vi "aggregator - v - real.vi"(8 "number":dbl, 10 "init?":bool, 11 "requested size":i32=20) -> (1 "Array":dbl[](array[numeric]))   [LabVIEW 2015]
uses:
  agregator -- action.ctl
  linear interpolation - real.vi
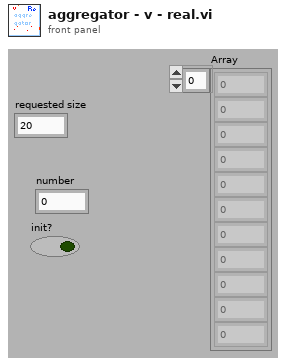
[diagram p1: front panel]
types:
  T1 = typedef "agregator -- action.ctl" = enum16{"append", "interpolate", "empty!", "force"}
  T2 = typedef "interpolation state - real.ctl" = cluster{"requested size":i32, "Array":dbl[], "actual number of elements":i32}
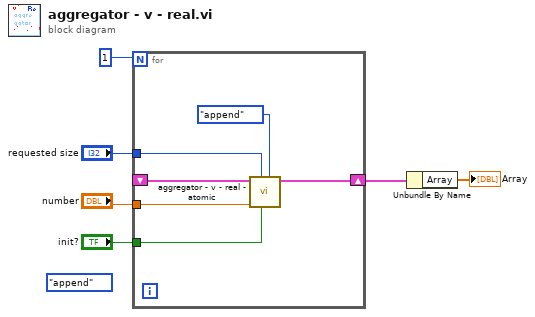
[diagram p0: block diagram]
diagram:
  (unwired) agregator_--_action."append" ("aggregator action")
  n1 = for {
    N: 1 -> [_]
    tunnel: "requested size" -> [w12]
    tunnel: "number" -> [w11]
    tunnel: "init?" -> [w10]
    shift-right: [w9] -> w2
    shift-left: _ -> [w8]
    n2 = call "aggregator - v - real - atomic.vi"("aggregator action"=agregator_--_action."append", "init?"=w10, "requested size"=w12, "number"=w11, "state IN"=w8) -> ("state OUT"=w9:T2)  [unwired: 3 in, 3 out]
  }
  n3 = Unbundle By Name(w2) -> ("Array"=→"Array":dbl[])
